vi "smooth_derivative.vi"(10 "Output Waveform":waveform(dbl), 11 "frequency":dbl) -> (3 "Filtered Signal":dynamicdata(waveform))   [LabVIEW 2019]
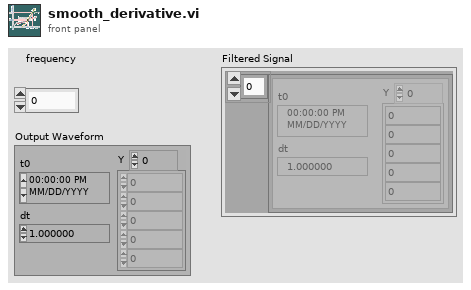
[diagram p1: front panel]
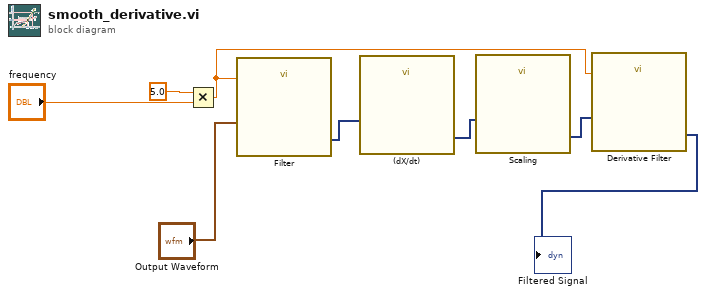
[diagram p0: block diagram]
diagram:
  n1 = Multiply(x=5.0, y="frequency") -> (x*y=w6:dbl)
  n2 = call "Filter"("Lower Cut-Off"=w6, "Signal"="Output Waveform") -> ("Filtered Signal"=w2:dynamicdata)  [unwired: 8 in, 1 out]
  n3 = call "(dX/dt)"("Signals"=w2) -> ("Result"=w3:dynamicdata)  [unwired: 5 in, 1 out]
  n4 = call "Scaling"("Signals"=w3) -> ("Scaled Signals"=w8:dynamicdata)  [unwired: 9 in, 1 out]
  n5 = call "Derivative Filter"("Lower Cut-Off"=w6, "Signal"=w8) -> ("Filtered Signal"=→"Filtered Signal":dynamicdata)  [unwired: 8 in, 1 out]
